vi "Timer.vi"(7 "Operation":enum16{"Start Timer", "Read Timing"}(ring)) -> (2 "Elapsed time":dbl)   [LabVIEW 2025]
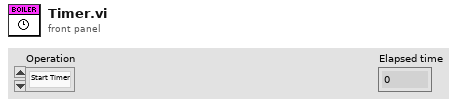
[diagram p1: front panel]
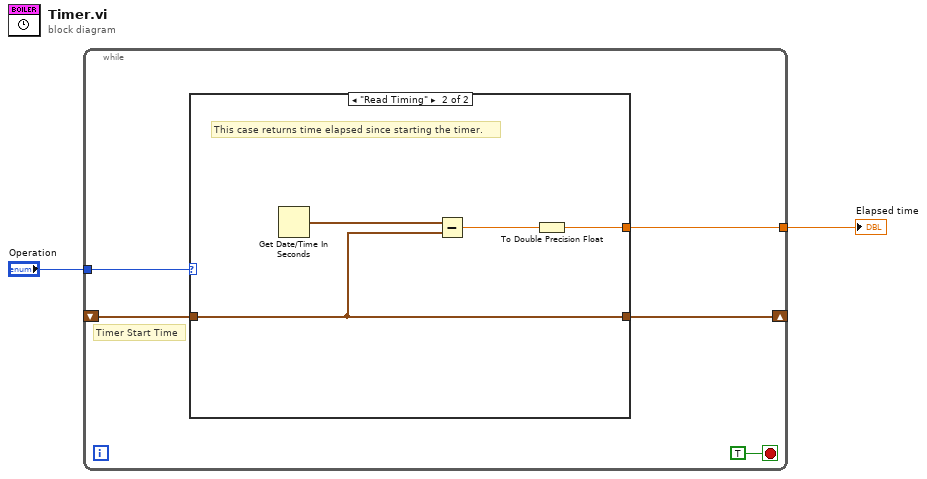
[diagram p0: block diagram]
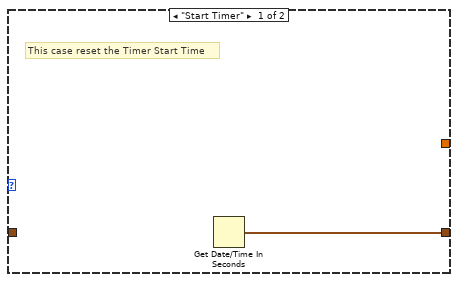
[diagram p2: hidden frame]
diagram:
  n1 = while {
    tunnel: "Operation" -> [w7]
    shift-right: [w6] -> _
    shift-left: _ -> [w5]
    tunnel: [w4] -> w1
    stop <- TRUE stop-if-true
    # "Timer Start Time"
    n2 = case shown="\"Read Timing\"" w7 {
      tunnel: [w8 w9] -> w6
      tunnel: w5 -> [_ w9]
      tunnel: [_ w10] -> w4
      frame "Start Timer" {
        # "This case reset the Timer Start Time"
        n3 = Get Date/Time In Seconds() -> (seconds since 1Jan1904=w8:timestamp)
      }
      frame "Read Timing" {
        # "This case returns time elapsed since starting the timer."
        n4 = Get Date/Time In Seconds() -> (seconds since 1Jan1904=w12:timestamp)
        n5 = Subtract(x=w12, y=w9) -> (x-y=w11:dbl)
        n6 = To Double Precision Float(number=w11) -> (double precision float=w10:dbl)
      }
    }
  }
  "Elapsed time" <- w1
